vi "Sensor_data_signed_unsigned_conv.vi"(0 "Datagram data":u16, 1 "sensor type":u8) -> (6 "Sensor raw value":i32)   [LabVIEW 2013]
doc: "force to wait data flow through error cluster for set value in ms. \nIf status message wired (not \"XXX\"), sends status message to global variable"
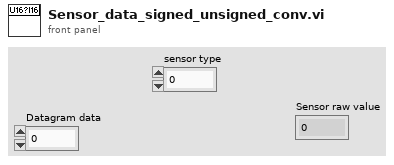
[diagram p1: front panel]
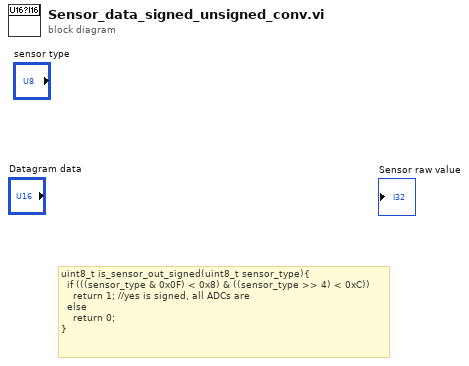
[diagram p0: block diagram]
diagram:
  # "uint8_t is_sensor_out_signed(uint8_t sensor_type){\n  if (((sensor_type & 0x0F) < 0x8) & ((sensor_type >> 4) < 0xC))\n    return 1; //yes is signed, all ADCs are\n  else\n    return 0;\n}"
